vi "AIT 664 - Create Sysdef Tree from DB Bus Configuration.vi"(0 "Section Ref in":T9 format="%.0x", 1 "Called From SysDef API (F)":bool, 5 "664 Device":T1, 11 "error in":errorcluster) -> (4 "Section Ref out":T9 format="%.0x", 6 "Item Ref":T9 format="%.0x", 15 "error out":errorcluster)   [LabVIEW 2013, in "AIT 664 Custom Device.lvlib"]
uses:
  AIT 664 Custom Device.lvlib
  <vilib>/NI Veristand/Custom Device API/Custom Device Item Ref.ctl
  Controls/664 - XML Device Description.ctl
  Controls/664 - XML End System Description.ctl
  Controls/664 - XML Output VL.ctl
  Controls/664 - XML Tx Message Port.ctl
  Controls/664 - Sampling Type.ctl
  Controls/664 -Param.ctl
  Controls/664 - XML Input VL.ctl
  Controls/664 - XML Rx Message Port.ctl
  Controls and Global/Global.vi
  <vilib>/NI Veristand/Custom Device API/Set Item Property (String).vi
  <vilib>/NI Veristand/Custom Device API/Custom Device API.lvlib
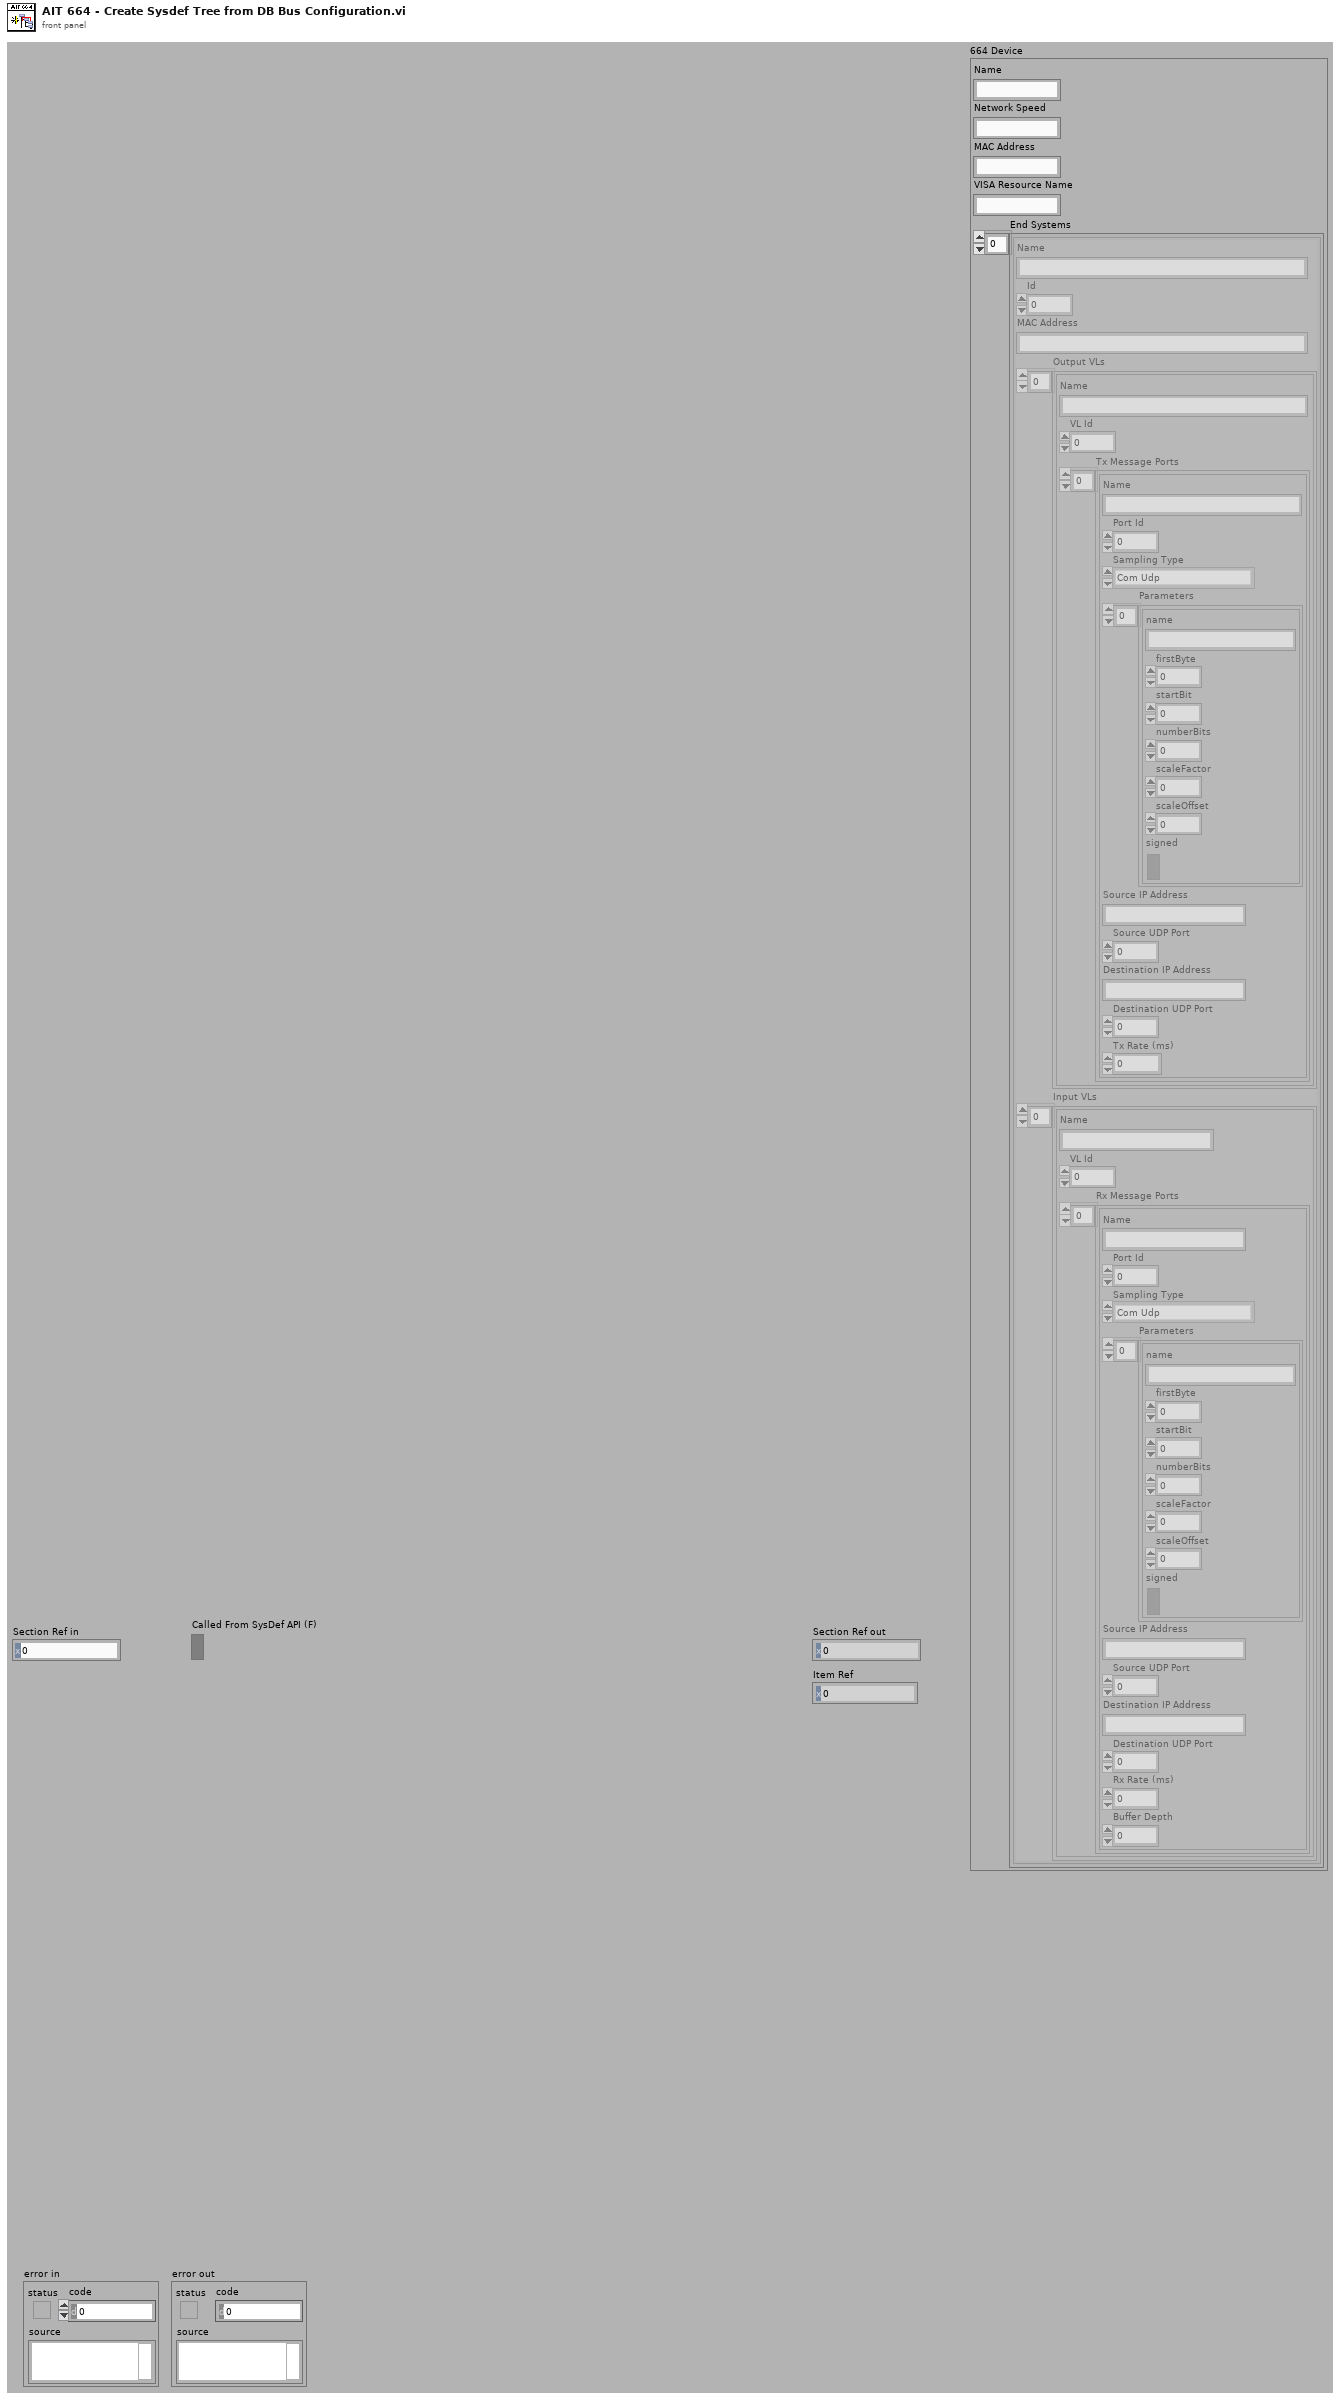
[diagram p1: front panel]
types:
  T1 = typedef "AIT 664 Custom Device.lvlib/664 - XML Device Description.ctl" = cluster{"Name":string, "Network Speed":string, "MAC Address":string, "VISA Resource Name":string, "End Systems":T2[]}
  T2 = typedef "AIT 664 Custom Device.lvlib/664 - XML End System Description.ctl" = cluster{"Name":string, "Id":u32, "MAC Address":string, "Output VLs":T3[], "Input VLs":T7[]}
  T3 = typedef "AIT 664 Custom Device.lvlib/664 - XML Output VL.ctl" = cluster{"Name":string, "VL Id":u32, "Tx Message Ports":T4[]}
  T4 = typedef "AIT 664 Custom Device.lvlib/664 - XML Tx Message Port.ctl" = cluster{"Name":string, "Port Id":u32, "Sampling Type":T5, "Parameters":T6[], "Source IP Address":string, "Source UDP Port":u32, "Destination IP Address":string, "Destination UDP Port":u32, "Tx Rate (ms)":u32}
  T5 = typedef "AIT 664 Custom Device.lvlib/664 - Sampling Type.ctl" = enum16{"Com Udp", "Com Udp Queuing", "Sap Udp", "Sap Ip", "Sap Mac", "Unknown"}
  T6 = typedef "AIT 664 Custom Device.lvlib/664 -Param.ctl" = cluster{"name":string, "firstByte":i32, "startBit":i32, "numberBits":i32, "scaleFactor":dbl, "scaleOffset":dbl, "signed":bool}
  T7 = typedef "AIT 664 Custom Device.lvlib/664 - XML Input VL.ctl" = cluster{"Name":string, "VL Id":u32, "Rx Message Ports":T8[]}
  T8 = typedef "AIT 664 Custom Device.lvlib/664 - XML Rx Message Port.ctl" = cluster{"Name":string, "Port Id":u32, "Sampling Type":T5, "Parameters":T6[], "Source IP Address":string, "Source UDP Port":u32, "Destination IP Address":string, "Destination UDP Port":u32, "Rx Rate (ms)":u32, "Buffer Depth":u32}
  T9 = typedef "Custom Device API.lvlib/Custom Device Item Ref.ctl" = u64
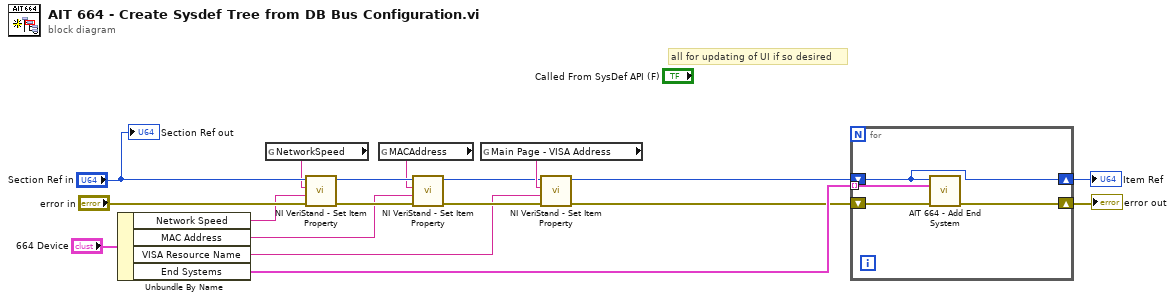
[diagram p0: block diagram]
diagram:
  # "all for updating of UI if so desired"
  n1 = Unbundle By Name("664 Device") -> ("Network Speed"=w14:string, "MAC Address"=w9:string, "VISA Resource Name"=w4:string, "End Systems"=w8:T2[])
  n2 = global read "Global.vi" "NetworkSpeed"() -> (w13:string)
  n3 = call-poly <vilib>:"NI VeriStand - Set Item Property.vi"("error in (no error)"="error in", "Value"=w14, "Property Name"=w13, "Item Ref in"="Section Ref in") -> ("error out"=w12:errorcluster, "Item Ref out"=w11:T9)  [unwired: 5 in, 1 out]
  n4 = global read "Global.vi" "MACAddress"() -> (w10:string)
  n5 = call-poly <vilib>:"NI VeriStand - Set Item Property.vi"("error in (no error)"=w12, "Value"=w9, "Property Name"=w10, "Item Ref in"=w11) -> ("error out"=w5:errorcluster, "Item Ref out"=w6:T9)  [unwired: 5 in, 1 out]
  n6 = global read "Global.vi" "Main Page - VISA Address"() -> (w7:string)
  n7 = call-poly <vilib>:"NI VeriStand - Set Item Property.vi"("error in (no error)"=w5, "Value"=w4, "Property Name"=w7, "Item Ref in"=w6) -> ("error out"=w2:errorcluster, "Item Ref out"=w3:T9)  [unwired: 5 in, 1 out]
  n8 = for {
    tunnel: w8 -> [w20] mode=indexing
    shift-right: [w22] -> w16
    shift-left: w2 -> [w21]
    shift-right: [w19] -> w1
    shift-left: w3 -> [w19]
    n9 = call "AIT 664 - Add End System.vi"("Node Ptr"=w19, "664 End System"=w20, "error in (no error)"=w21) -> ("error out"=w22:errorcluster)  [unwired: 11 in, 1 out]
  }
  "error out" <- w16
  "Item Ref" <- w1
  "Section Ref out" <- "Section Ref in"
